vi "Write XY Graph.vi"(8 "error in (no error)":errorcluster, 10 "XY Graph":cluster{dbl[], dbl[]}[](array[cluster]), 11 "GarphView in":refnum<class "GarphView.lvclass">) -> (0 "error out":errorcluster, 3 "GarphView out":refnum<class "GarphView.lvclass">)   [LabVIEW 2020, in "GarphView.lvlib" / "GarphView.lvclass"]
uses:
  GarphView.lvclass
  GarphView.lvclass/GarphView.ctl
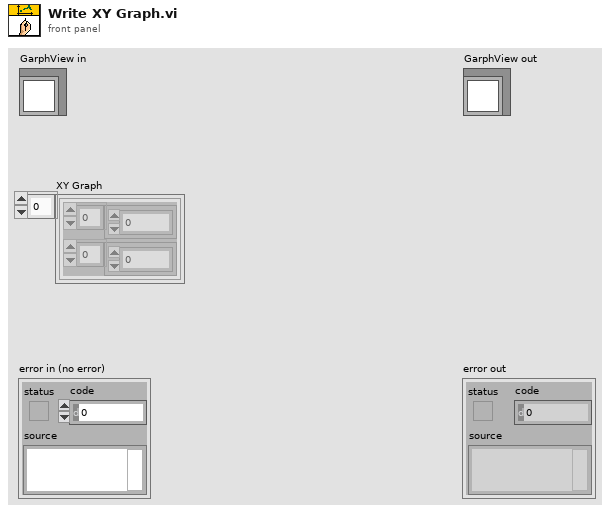
[diagram p1: front panel]
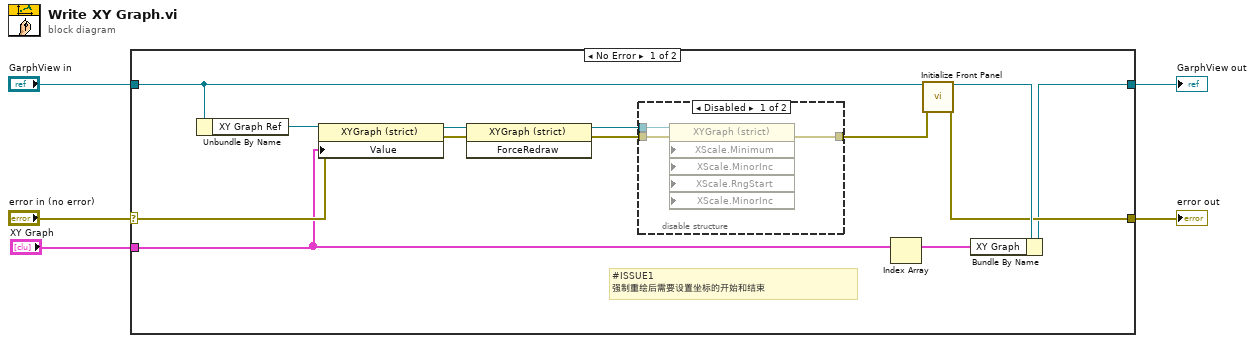
[diagram p0: block diagram]
diagram:
  n1 = case shown="No Error" "error in (no error)" {
    selector: "error in (no error)" -> [w17 w24]
    tunnel: [w13 w24] -> w4
    tunnel: [w12 w23] -> w2
    tunnel: "GarphView in" -> [w16 w23]
    tunnel: "XY Graph" -> [w11 _]
    frame No Error {
      # "#ISSUE1\n强制重绘后需要设置坐标的开始和结束"
      n2 = Unbundle By Name(w16) -> ("XY Graph Ref"=w18:refnum<vi>)
      n3 = property class="XYGraph (strict)"(reference=w18, error in=w17, "Value"=w11) -> (reference out=w9:refnum<vi>, error out=w14:errorcluster)
      n4 = invoke class="XYGraph (strict)" method="ForceRedraw"(reference=w9, error in=w14) -> (reference out=w8:refnum<vi>, error out=w7:errorcluster)  [unwired: 1 in, 1 out]
      n5 = disable-structure shown="Disabled" {
        disable-tunnel: w8 -> [w21 _]
        disable-tunnel: w7 -> [w20 w22]
        disable-tunnel: [w19 w22] -> w6
        frame Disabled {
          n6 = property class="XYGraph (strict)" props=["XScale", "Minimum", "XScale", "MinorInc", "XScale", "RngStart", "XScale", "MinorInc"](reference=w21, error in=w20) -> (error out=w19:errorcluster)  [unwired: 4 in, 1 out]
        }
        frame Enabled {
        }
      }
      n7 = Index Array(array=w11) -> (element=w10:cluster{dbl[], dbl[]})  [unwired: 1 in]
      n8 = call-dynamic "Initialize Front Panel.vi"("error in (no error)"=w6, "GarphView in"=w16) -> ("error out"=w13:errorcluster, "GarphView out"=w15:refnum<class "GarphView.lvclass">)  [unwired: 8 in]
      n9 = Bundle By Name(cluster=w15, "XY Graph"=w10) -> (w12:refnum<class "GarphView.lvclass">)
    }
    frame Error {
    }
  }
  "error out" <- w4
  "GarphView out" <- w2
